vi "LSMcontroller_v63_3Dfocus.vi"() -> ()   [LabVIEW 2015] (continued)
                                n2570 = Bundle By Name(cluster=w5649, "AO"=w5648, "E_AO"=w5647) -> (w5646:T25)
                                n2571 = call "tempconfigAO.vi"("Temp Config in"=w5646, "command"="set") -> ()  [unwired: 1 out]
                                }
                                frame #1 {
                                n2572 = call "tempconfigAI.vi"("command"="get") -> ("Temp Config out"=w5661:T26)  [unwired: 1 in]
                                n2573 = Unbundle By Name(w5661) -> ("AI"=w5666:refnum<k21>, "E_AI"=w5667:errorcluster)
                                n2574 = call <vilib>:"DAQmx Start Task.vi"("task/channels in"=w5666, "error in"=w5667) -> ("task out"=w5668:refnum<k21>, "error out"=w5669:errorcluster)  [unwired: 12 in]
                                n2575 = call "tempconfigAI.vi"("command"="get") -> ("Temp Config out"=w5663:T26)  [unwired: 1 in]
                                n2576 = Bundle By Name(cluster=w5663, "AI"=w5668, "E_AI"=w5669) -> (w5665:T26)
                                n2577 = call "tempconfigAI.vi"("Temp Config in"=w5665, "command"="set") -> ()  [unwired: 1 out]
                                }
                                }
                                }
                              }
                              n2578 = case shown="True" w5645 {
                                frame False {
                                }
                                frame True {
                                n2579 = local write "set as Rp?"(FALSE ("set as Rp?")) -> ()
                                }
                              }
                            }
                          }
                        }
                        frame True {
                        }
                      }
                      n2580 = local read "sealtest"() -> (w5526:bool)
                      n2581 = Not(x=w5526) -> (.not. x?=w5525:bool)
                    }
                  }
                  frame #4 {
                    n2582 = call "tempconfigAO.vi"("command"="get") -> ("Temp Config out"=w5696:T25)  [unwired: 1 in]
                    n2583 = Unbundle By Name(w5696) -> ("AO"=w5695:refnum<k21>[], "E_AO"=w5694:errorcluster[])
                    n2584 = call "configuration.vi"("command"="get") -> ("config out"=w5677:T11)  [unwired: 2 in, 1 out]
                    n2585 = call "tempconfigAI.vi"("command"="get") -> ("Temp Config out"=w5683:T26)  [unwired: 1 in]
                    n2586 = Unbundle By Name(w5677) -> ("Device 1 sampleclock out"=w5674:tag, "Device 1 Starttrigger out"=w5673:tag)
                    n2587 = Unbundle By Name(w5683) -> ("AI"=w5684:refnum<k21>, "E_AI"=w5685:errorcluster)
                    n2588 = for {
                      tunnel: w5695 -> [w5700] mode=indexing
                      tunnel: w5694 -> [w5699] mode=indexing
                      tunnel: [w5698] -> w5690 mode=indexing
                      n2589 = call <vilib>:"DAQmx Stop Task.vi"("task/channels in"=w5700, "error in"=w5699) -> ("task out"=w5701:refnum<k21>, "error out"=w5702:errorcluster)  [unwired: 12 in]
                      n2590 = call <vilib>:"DAQmx Clear Task.vi"("task in"=w5701, "error in"=w5702) -> ("error out"=w5698:errorcluster)  [unwired: 13 in]
                    }
                    n2591 = call <vilib>:"DAQmx Stop Task.vi"("task/channels in"=w5684, "error in"=w5685) -> ("task out"=w5681:refnum<k21>, "error out"=w5680:errorcluster)  [unwired: 12 in]
                    n2592 = call <vilib>:"DAQmx Disconnect Terminals.vi"("source terminal"=tag "/Dev1/ai/SampleClock", "destination terminal"=w5674) -> ("error out"=w5671:errorcluster)  [unwired: 13 in]
                    n2593 = call <vilib>:"DAQmx Clear Task.vi"("task in"=w5681, "error in"=w5680) -> ("error out"=w5679:errorcluster)  [unwired: 13 in]
                    n2594 = call "tempconfigAO.vi"("command"="get") -> ("Temp Config out"=w5691:T25)  [unwired: 1 in]
                    n2595 = Bundle By Name(cluster=w5691, "E_AO"=w5690) -> (w5689:T25)
                    n2596 = call "tempconfigAI.vi"("command"="get") -> ("Temp Config out"=w5687:T26)  [unwired: 1 in]
                    n2597 = Bundle By Name(cluster=w5687, "E_AI"=w5679) -> (w5678:T26)
                    n2598 = call "tempconfigAO.vi"("Temp Config in"=w5689, "command"="set") -> ()  [unwired: 1 out]
                    n2599 = call <vilib>:"DAQmx Disconnect Terminals.vi"("source terminal"=tag "/Dev1/ai/StartTrigger", "destination terminal"=w5673, "error in"=w5671) -> ()  [unwired: 12 in, 1 out]
                    n2600 = call "tempconfigAI.vi"("Temp Config in"=w5678, "command"="set") -> ()  [unwired: 1 out]
                  }
                  frame #5 {
                    w5705 = T21 4 items=["no dialog", "OK message", "continue or stop message", "OK message + warnings", "continue/stop + warnings"] ("type of dialog (OK msg:1)")
                    n2601 = call "displayerrors.vi"() -> ("error IO"=w5704:errorcluster)
                    n2602 = call "zeropatch.vi"() -> ()  [unwired: 12 in]
                    n2603 = call <vilib>:"Simple Error Handler.vi"("type of dialog (OK msg:1)"=w5705, "error in (no error)"=w5704) -> ("error out"=w5703:errorcluster)  [unwired: 3 in, 4 out]
                    n2604 = call <vilib>:"Clear Errors.vi"("error in (no error)"=w5703) -> ()  [unwired: 5 in, 2 out]
                  }
                }
              }
            }
          }
          event "readpatch": Value Change {
            n2605 = event-data() -> ()  [unwired: 1 in, 6 out]
            n2606 = local read "readpatch"() -> (w5706:bool)
            n2607 = case shown="True" w5706 {
              frame False {
              }
              frame True {
                n2608 = stacked-sequence {
                  seq-local: [w5707 _ _ _ _ _] -> [_ w5740 _ w5792 _ _]
                  frame #0 {
                    n2609 = stacked-sequence {
                      tunnel: [_ w5719 _] -> w5707
                      frame #0 {
                        n2610 = call "2pparameters.vi"("command"="get") -> ("params out"=w5712:T10)  [unwired: 1 in]
                        n2611 = Unbundle By Name(w5712) -> ("autoshutter"=w5713:bool)
                        n2612 = local read "OCchecked?"() -> (w5710:bool)
                        n2613 = call "sealtestwfparams.vi"("command"="set") -> ()  [unwired: 6 in, 1 out]
                        n2614 = case shown="False" w5710 {
                          frame False {
                            n2615 = One Button Dialog(message="Is the OC gain correct?", button name ("OK")="ok") -> (true=w5714:bool)
                            n2616 = local write "OCchecked?"(w5714) -> ()
                          }
                          frame True {
                          }
                        }
                        n2617 = case shown="True" w5713 {
                          frame False {
                          }
                          frame True {
                            n2618 = call "shuttercontrol.vi"("command"="close") -> ()  [unwired: 1 in, 1 out]
                          }
                        }
                        n2619 = call "allAI-temp.vi"("command"=enum16{"get", "set", "clear", "append"}."clear") -> ()  [unwired: 3 in, 2 out]
                      }
                      frame #1 {
                        n2620 = call "sealtestwfparams.vi"("command"="get") -> ("Params out"=w5725:T22)  [unwired: 6 in]
                        n2621 = Unbundle By Name(w5725) -> ("AO parameters"=w5723:T23)
                        n2622 = Index Array(array=w5723, index=1) -> (element=w5722:T24)
                        n2623 = call "generateRampedSquareWave_fromAOparameters.vi"("AO params"=w5722) -> ("Waveform"=w5718:waveform(dbl), "wflength"=w5719:i32)
                        n2624 = Build Array(w5718) -> (w5721:waveform(dbl)[])
                        n2625 = call "waveformssealtestbuffer.vi"("AO wf in"=w5721, "command"="set") -> ()  [unwired: 1 out]
                      }
                      frame #2 {
                        n2626 = local read "Vholding (mV)"() -> (w5728:sgl)
                        n2627 = local read "Current Clamp"() -> (w5734:bool)
                        n2628 = local read "Voltage Clamp"() -> (w5733:bool)
                        n2629 = local read "OCgain"() -> (w5729:sgl)
                        n2630 = local read "CC_ICgain"() -> (w5732:dbl)
                        n2631 = local read "holdon"() -> (w5727:bool)
                        n2632 = call "patchparameters.vi"("command"="get") -> ("Params out"=w5736:T13)  [unwired: 1 in]
                        n2633 = Bundle By Name(cluster=w5736, "VC"=w5733, "CC"=w5734, "CC_icg (pA/mv)"=w5732, "VC_icg (mV/mV)"=10.0, "OCG (mV/pA)"=w5729, "OVG (mV/mV)"=0.1, "Vhold (mV)"=w5728, "holdon"=w5727) -> (w5735:T13)
                        n2634 = call "patchparameters.vi"("Params in"=w5735, "command"="set") -> ()  [unwired: 1 out]
                      }
                    }
                  }
                  frame #1 {
                    w5739 = 2
                    n2635 = call "patchparameters.vi"("command"="get") -> ("Params out"=w5747:T13)  [unwired: 1 in]
                    n2636 = Unbundle By Name(w5747) -> ("holdon"=w5746:bool, "Vhold (mV)"=w5745:sgl, "CC_icg (pA/mv)"=w5753:sgl, "CC"=w5751:bool, "VC_icg (mV/mV)"=w5752:sgl)
                    n2637 = Select(t=w5753, s=w5751, f=w5752) -> (s? t:f=w5754:sgl)
                    n2638 = To Single Precision Float(number=0.001 ("y")) -> (single precision float=w5755:sgl)
                    n2639 = Compound Arithmetic op=MULTIPLY(w5745, w5754, w5755) -> (w5749:sgl)
                    n2640 = case shown="False" w5746 {
                      tunnel: w5749 -> [_ w5767]
                      tunnel: [0.0 w5767] -> w5742
                      frame False {
                      }
                      frame True {
                      }
                    }
                    n2641 = Greater Than 0?(x=w5739) -> (x > 0?=w5741:bool)
                    n2642 = case shown="True" w5741 {
                      tunnel: w5740 -> [_ w5756]
                      tunnel: w5739 -> [_ w5759]
                      frame False {
                      }
                      frame True {
                        n2643 = Initialize Array(sgl 0.0 ("element"), w5759, w5756) -> (w5757:sgl[][])
                        n2644 = call "allAI-temp.vi"("array in"=w5757, "command"=enum16{"get", "set", "clear", "append"}."set") -> ()  [unwired: 2 in, 2 out]
                      }
                    }
                    n2645 = flat-sequence {
                      tunnel: w5740 -> [w5763]
                      tunnel: w5740 -> [w5762]
                      tunnel: [w5762] -> w5744
                      tunnel: [w5761] -> w5743
                      tunnel: w5742 -> [w5761]
                      tunnel: w5744 -> [w5765]
                      tunnel: w5743 -> [w5764]
                      frame #0 {
                        n2646 = call "prepAI_sealtest.vi"("samples per channel"=w5763) -> ()  [unwired: 2 in]
                      }
                      frame #1 {
                        n2647 = call "prepAO_sealtest.vi"("Vhold"=w5764, "samples per channel"=w5765) -> ()  [unwired: 1 in]
                      }
                    }
                  }
                  frame #2 {
                    n2648 = stacked-sequence {
                      frame #0 {
                        n2649 = call "tempconfigAO.vi"("command"="get") -> ("Temp Config out"=w5771:T25)  [unwired: 1 in]
                        n2650 = Unbundle By Name(w5771) -> ("AO"=w5772:refnum<k21>[], "E_AO"=w5773:errorcluster[])
                        n2651 = for {
                          tunnel: w5772 -> [w5781] mode=indexing
                          tunnel: w5773 -> [w5780] mode=indexing
                          tunnel: [w5779] -> w5775 mode=indexing
                          tunnel: [w5778] -> w5776 mode=indexing
                          n2652 = call <vilib>:"DAQmx Start Task.vi"("task/channels in"=w5781, "error in"=w5780) -> ("task out"=w5779:refnum<k21>, "error out"=w5778:errorcluster)  [unwired: 12 in]
                        }
                        n2653 = call "tempconfigAO.vi"("command"="get") -> ("Temp Config out"=w5774:T25)  [unwired: 1 in]
                        n2654 = Bundle By Name(cluster=w5774, "AO"=w5775, "E_AO"=w5776) -> (w5777:T25)
                        n2655 = call "tempconfigAO.vi"("Temp Config in"=w5777, "command"="set") -> ()  [unwired: 1 out]
                      }
                      frame #1 {
                        n2656 = call "tempconfigAI.vi"("command"="get") -> ("Temp Config out"=w5783:T26)  [unwired: 1 in]
                        n2657 = Unbundle By Name(w5783) -> ("AI"=w5788:refnum<k21>, "E_AI"=w5789:errorcluster)
                        n2658 = call <vilib>:"DAQmx Start Task.vi"("task/channels in"=w5788, "error in"=w5789) -> ("task out"=w5790:refnum<k21>, "error out"=w5791:errorcluster)  [unwired: 12 in]
                        n2659 = call "tempconfigAI.vi"("command"="get") -> ("Temp Config out"=w5785:T26)  [unwired: 1 in]
                        n2660 = Bundle By Name(cluster=w5785, "AI"=w5790, "E_AI"=w5791) -> (w5787:T26)
                        n2661 = call "tempconfigAI.vi"("Temp Config in"=w5787, "command"="set") -> ()  [unwired: 1 out]
                      }
                    }
                  }
                  frame #3 {
                    n2662 = while {
                      tunnel: w5792 -> [w5793]
                      stop <- w5794 stop-if-true
                      n2663 = local read "readpatch"() -> (w5797:bool)
                      n2664 = Not(x=w5797) -> (.not. x?=w5796:bool)
                      n2665 = case shown="True" w5796 {
                        tunnel: w5793 -> [w5798 _]
                        frame False {
                          n2666 = stacked-sequence {
                            seq-local: [w5799 _ _ _ _ _] -> [_ w5808 _ w5831 w5878 w5897]
                            tunnel: w5798 -> [_ _ w5816 _ w5877 _]
                            frame #0 {
                              n2667 = call "patchparameters.vi"("command"="get") -> ("Params out"=w5806:T13)  [unwired: 1 in]
                              n2668 = local read "Vholding (mV)"() -> (w5803:sgl)
                              n2669 = Unbundle By Name(w5806) -> ("Vhold (mV)"=w5802:sgl, "holdon"=w5805:bool)
                              n2670 = local read "holdon"() -> (w5804:bool)
                              n2671 = Not Equal?(x=w5803, y=w5802) -> (x != y?=w5801:bool)
                              n2672 = Not Equal?(x=w5805, y=w5804) -> (x != y?=w5800:bool)
                              n2673 = Or(x=w5801, y=w5800) -> (x .or. y?=w5799:bool)
                            }
                            frame #1 {
                              n2674 = case shown="False" w5808 {
                                frame False {
                                }
                                frame True {
                                n2675 = local read "Vholding (mV)"() -> (w5811:sgl)
                                n2676 = local read "holdon"() -> (w5809:bool)
                                n2677 = call "patchparameters.vi"("command"="get") -> ("Params out"=w5812:T13)  [unwired: 1 in]
                                n2678 = Bundle By Name(cluster=w5812, "Vhold (mV)"=w5811, "holdon"=w5809) -> (w5810:T13)
                                n2679 = call "patchparameters.vi"("Params in"=w5810, "command"="set") -> ()  [unwired: 1 out]
                                }
                              }
                            }
                            frame #2 {
                              n2680 = call "tempconfigAI.vi"("command"="get") -> ("Temp Config out"=w5826:T26)  [unwired: 1 in]
                              n2681 = Unbundle By Name(w5826) -> ("AI"=w5825:refnum<k21>, "E_AI"=w5824:errorcluster)
                              n2682 = call-poly <vilib>:"DAQmx Read.vi"("task/channels in"=w5825, "number of samples per channel"=w5816, "timeout"=10.0, "error in"=w5824) -> ("task out"=w5820:refnum<k21>, "data"=w5817:i16[][], "error out"=w5829:errorcluster)  [unwired: 9 in]
                              n2683 = call "tempconfigAI.vi"("command"="get") -> ("Temp Config out"=w5821:T26)  [unwired: 1 in]
                              n2684 = Bundle By Name(cluster=w5821, "AI"=w5820, "E_AI"=w5829) -> (w5828:T26)
                              n2685 = To Single Precision Float(number=w5817) -> (single precision float=w5819:sgl[][])
                              n2686 = call "tempconfigAI.vi"("Temp Config in"=w5828, "command"="set") -> ()  [unwired: 1 out]
                              n2687 = call "allAI-temp.vi"("array in"=w5819, "command"=enum16{"get", "set", "clear", "append"}."set") -> ()  [unwired: 2 in, 2 out]
                            }
                            frame #3 {
                              n2688 = case shown="True" w5831 {
                                frame False {
                                }
                                frame True {
                                n2689 = call "tempconfigAO.vi"("command"="get") -> ("Temp Config out"=w5870:T25)  [unwired: 1 in]
                                n2690 = Unbundle By Name(w5870) -> ("AO"=w5869:refnum<k21>[], "E_AO"=w5868:errorcluster[])
                                n2691 = call "tempconfigAI.vi"("command"="get") -> ("Temp Config out"=w5857:T26)  [unwired: 1 in]
                                n2692 = Unbundle By Name(w5857) -> ("AI"=w5858:refnum<k21>, "E_AI"=w5859:errorcluster)
                                n2693 = for {
                                tunnel: w5869 -> [w5874] mode=indexing
                                tunnel: w5868 -> [w5873] mode=indexing
                                tunnel: [w5872] -> w5864 mode=indexing
                                n2694 = call <vilib>:"DAQmx Stop Task.vi"("task/channels in"=w5874, "error in"=w5873) -> ("task out"=w5875:refnum<k21>, "error out"=w5876:errorcluster)  [unwired: 12 in]
                                n2695 = call <vilib>:"DAQmx Clear Task.vi"("task in"=w5875, "error in"=w5876) -> ("error out"=w5872:errorcluster)  [unwired: 13 in]
                                }
                                n2696 = call <vilib>:"DAQmx Stop Task.vi"("task/channels in"=w5858, "error in"=w5859) -> ("task out"=w5855:refnum<k21>, "error out"=w5854:errorcluster)  [unwired: 12 in]
                                n2697 = call <vilib>:"DAQmx Clear Task.vi"("task in"=w5855, "error in"=w5854) -> ("error out"=w5853:errorcluster)  [unwired: 13 in]
                                n2698 = call "tempconfigAO.vi"("command"="get") -> ("Temp Config out"=w5865:T25)  [unwired: 1 in]
                                n2699 = Bundle By Name(cluster=w5865, "E_AO"=w5864) -> (w5863:T25)
                                n2700 = call "tempconfigAI.vi"("command"="get") -> ("Temp Config out"=w5861:T26)  [unwired: 1 in]
                                n2701 = Bundle By Name(cluster=w5861, "E_AI"=w5853) -> (w5852:T26)
                                n2702 = call "tempconfigAO.vi"("Temp Config in"=w5863, "command"="set") -> ()  [unwired: 1 out]
                                n2703 = call "tempconfigAI.vi"("Temp Config in"=w5852, "command"="set") -> ()  [unwired: 1 out]
                                }
                              }
                              n2704 = call "allAI-temp.vi"("command"=enum16{"get", "set", "clear", "append"}."get") -> ("array out"=w5835:sgl[][])  [unwired: 3 in, 1 out]
                              n2705 = call "tempconfigAI.vi"("command"="get") -> ("Temp Config out"=w5847:T26)  [unwired: 1 in]
                              n2706 = call "tempconfigAI.vi"("command"="get") -> ("Temp Config out"=w5849:T26)  [unwired: 1 in]
                              n2707 = Unbundle By Name(w5847) -> ("header"=w5845:dbl[])
                              n2708 = Unbundle By Name(w5849) -> ("header"=w5851:dbl[])
                              n2709 = Index Array(array=w5835, index (row) #1=1 ("index (row)"), index (row) #2=0 ("index (row)")) -> (element #1=w5833:sgl[], element #2=w5832:sgl[])  [unwired: 2 in]
                              n2710 = local read "OCgain"() -> (w5839:sgl)
                              n2711 = call "Unscaledtoscaled.vi"("Unscaled Data"=w5833, "Header Information"=w5845) -> ("Array"=w5844:sgl[])  [unwired: 1 in]
                              n2712 = call "Unscaledtoscaled.vi"("Unscaled Data"=w5832, "Header Information"=w5851) -> ("Array"=w5848:sgl[])  [unwired: 1 in]
                              n2713 = Multiply(x=w5844, y=0.1) -> (x*y=w5841:dbl[])
                              n2714 = Divide(x=w5848, y=w5839) -> (x/y=w5840:sgl[])
                              n2715 = Build Array(w5841, w5840) -> (w5843:dbl[][])
                              n2716 = Multiply(x=w5843, y=1000.0) -> (x*y=w5830:dbl[][])
                              n2717 = local write "Patch readout"(w5830) -> ()
                            }
                            frame #4 {
                              n2718 = case shown="True" w5878 {
                                tunnel: w5877 -> [_ w5879]
                                frame False {
                                }
                                frame True {
                                n2719 = call "patchparameters.vi"("command"="get") -> ("Params out"=w5883:T13)  [unwired: 1 in]
                                n2720 = Unbundle By Name(w5883) -> ("holdon"=w5882:bool, "Vhold (mV)"=w5881:sgl, "CC_icg (pA/mv)"=w5889:sgl, "CC"=w5887:bool, "VC_icg (mV/mV)"=w5888:sgl)
                                n2721 = Select(t=w5889, s=w5887, f=w5888) -> (s? t:f=w5890:sgl)
                                n2722 = To Single Precision Float(number=0.001 ("y")) -> (single precision float=w5891:sgl)
                                n2723 = Compound Arithmetic op=MULTIPLY(w5881, w5890, w5891) -> (w5885:sgl)
                                n2724 = case shown="True" w5882 {
                                tunnel: w5885 -> [_ w5896]
                                tunnel: [0.0 w5896] -> w5880
                                frame False {
                                }
                                frame True {
                                }
                                }
                                n2725 = flat-sequence {
                                tunnel: w5879 -> [w5892]
                                tunnel: w5880 -> [w5894]
                                tunnel: w5879 -> [w5893]
                                frame #0 {
                                n2726 = call "prepAI_sealtest.vi"("samples per channel"=w5892) -> ()  [unwired: 2 in]
                                }
                                frame #1 {
                                n2727 = call "prepAO_sealtest.vi"("Vhold"=w5894, "samples per channel"=w5893) -> ()  [unwired: 1 in]
                                }
                                }
                                }
                              }
                            }
                            frame #5 {
                              n2728 = case shown="True" w5897 {
                                frame False {
                                }
                                frame True {
                                n2729 = stacked-sequence {
                                frame #0 {
                                n2730 = call "tempconfigAO.vi"("command"="get") -> ("Temp Config out"=w5904:T25)  [unwired: 1 in]
                                n2731 = Unbundle By Name(w5904) -> ("AO"=w5903:refnum<k21>[], "E_AO"=w5902:errorcluster[])
                                n2732 = for {
                                tunnel: w5903 -> [w5911] mode=indexing
                                tunnel: w5902 -> [w5910] mode=indexing
                                tunnel: [w5909] -> w5900 mode=indexing
                                tunnel: [w5908] -> w5899 mode=indexing
                                n2733 = call <vilib>:"DAQmx Start Task.vi"("task/channels in"=w5911, "error in"=w5910) -> ("task out"=w5909:refnum<k21>, "error out"=w5908:errorcluster)  [unwired: 12 in]
                                }
                                n2734 = call "tempconfigAO.vi"("command"="get") -> ("Temp Config out"=w5901:T25)  [unwired: 1 in]
                                n2735 = Bundle By Name(cluster=w5901, "AO"=w5900, "E_AO"=w5899) -> (w5898:T25)
                                n2736 = call "tempconfigAO.vi"("Temp Config in"=w5898, "command"="set") -> ()  [unwired: 1 out]
                                }
                                frame #1 {
                                n2737 = call "tempconfigAI.vi"("command"="get") -> ("Temp Config out"=w5913:T26)  [unwired: 1 in]
                                n2738 = Unbundle By Name(w5913) -> ("AI"=w5918:refnum<k21>, "E_AI"=w5919:errorcluster)
                                n2739 = call <vilib>:"DAQmx Start Task.vi"("task/channels in"=w5918, "error in"=w5919) -> ("task out"=w5920:refnum<k21>, "error out"=w5921:errorcluster)  [unwired: 12 in]
                                n2740 = call "tempconfigAI.vi"("command"="get") -> ("Temp Config out"=w5915:T26)  [unwired: 1 in]
                                n2741 = Bundle By Name(cluster=w5915, "AI"=w5920, "E_AI"=w5921) -> (w5917:T26)
                                n2742 = call "tempconfigAI.vi"("Temp Config in"=w5917, "command"="set") -> ()  [unwired: 1 out]
                                }
                                }
                                }
                              }
                            }
                          }
                        }
                        frame True {
                        }
                      }
                      n2743 = local read "readpatch"() -> (w5795:bool)
                      n2744 = Not(x=w5795) -> (.not. x?=w5794:bool)
                    }
                  }
                  frame #4 {
                    n2745 = call "tempconfigAO.vi"("command"="get") -> ("Temp Config out"=w5947:T25)  [unwired: 1 in]
                    n2746 = Unbundle By Name(w5947) -> ("AO"=w5946:refnum<k21>[], "E_AO"=w5945:errorcluster[])
                    n2747 = call "configuration.vi"("command"="get") -> ("config out"=w5928:T11)  [unwired: 2 in, 1 out]
                    n2748 = call "tempconfigAI.vi"("command"="get") -> ("Temp Config out"=w5934:T26)  [unwired: 1 in]
                    n2749 = Unbundle By Name(w5928) -> ("Device 1 sampleclock out"=w5925:tag, "Device 1 Starttrigger out"=w5924:tag)
                    n2750 = Unbundle By Name(w5934) -> ("AI"=w5935:refnum<k21>, "E_AI"=w5936:errorcluster)
                    n2751 = for {
                      tunnel: w5946 -> [w5951] mode=indexing
                      tunnel: w5945 -> [w5950] mode=indexing
                      tunnel: [w5949] -> w5941 mode=indexing
                      n2752 = call <vilib>:"DAQmx Stop Task.vi"("task/channels in"=w5951, "error in"=w5950) -> ("task out"=w5952:refnum<k21>, "error out"=w5953:errorcluster)  [unwired: 12 in]
                      n2753 = call <vilib>:"DAQmx Clear Task.vi"("task in"=w5952, "error in"=w5953) -> ("error out"=w5949:errorcluster)  [unwired: 13 in]
                    }
                    n2754 = call <vilib>:"DAQmx Stop Task.vi"("task/channels in"=w5935, "error in"=w5936) -> ("task out"=w5932:refnum<k21>, "error out"=w5931:errorcluster)  [unwired: 12 in]
                    n2755 = call <vilib>:"DAQmx Disconnect Terminals.vi"("source terminal"=tag "/Dev1/ai/SampleClock", "destination terminal"=w5925) -> ("error out"=w5922:errorcluster)  [unwired: 13 in]
                    n2756 = call <vilib>:"DAQmx Clear Task.vi"("task in"=w5932, "error in"=w5931) -> ("error out"=w5930:errorcluster)  [unwired: 13 in]
                    n2757 = call "tempconfigAO.vi"("command"="get") -> ("Temp Config out"=w5942:T25)  [unwired: 1 in]
                    n2758 = Bundle By Name(cluster=w5942, "E_AO"=w5941) -> (w5940:T25)
                    n2759 = call "tempconfigAI.vi"("command"="get") -> ("Temp Config out"=w5938:T26)  [unwired: 1 in]
                    n2760 = Bundle By Name(cluster=w5938, "E_AI"=w5930) -> (w5929:T26)
                    n2761 = call "tempconfigAO.vi"("Temp Config in"=w5940, "command"="set") -> ()  [unwired: 1 out]
                    n2762 = call <vilib>:"DAQmx Disconnect Terminals.vi"("source terminal"=tag "/Dev1/ai/StartTrigger", "destination terminal"=w5924, "error in"=w5922) -> ()  [unwired: 12 in, 1 out]
                    n2763 = call "tempconfigAI.vi"("Temp Config in"=w5929, "command"="set") -> ()  [unwired: 1 out]
                  }
                  frame #5 {
                    w5956 = T21 4 items=["no dialog", "OK message", "continue or stop message", "OK message + warnings", "continue/stop + warnings"] ("type of dialog (OK msg:1)")
                    n2764 = call "displayerrors.vi"() -> ("error IO"=w5955:errorcluster)
                    n2765 = call "zeropatch.vi"() -> ()  [unwired: 12 in]
                    n2766 = call <vilib>:"Simple Error Handler.vi"("type of dialog (OK msg:1)"=w5956, "error in (no error)"=w5955) -> ("error out"=w5954:errorcluster)  [unwired: 3 in, 4 out]
                    n2767 = call <vilib>:"Clear Errors.vi"("error in (no error)"=w5954) -> ()  [unwired: 5 in, 2 out]
                  }
                }
              }
            }
          }
          event "Current Clamp": Value Change {
            n2768 = event-data() -> ()  [unwired: 1 in, 6 out]
            n2769 = local read "Current Clamp"() -> (w5961:bool)
            n2770 = property on="Vholding (mV)" class="DigNum (strict)"("Caption.Text"="Ihold (pA)") -> ()  [unwired: 2 in, 2 out]
            n2771 = Not(x=w5961) -> (.not. x?=w5960:bool)
            n2772 = property on="Voltage Clamp" class="Bool (strict)"("Value"=w5960) -> ()  [unwired: 2 in, 2 out]
            n2773 = One Button Dialog(message="Have you switched the HEKA to CC and changed the external input cable?", button name ("OK")="Ok") -> ()  [unwired: 1 out]
          }
          event "Voltage Clamp": Value Change {
            n2774 = event-data() -> ()  [unwired: 1 in, 6 out]
            n2775 = local read "Voltage Clamp"() -> (w5966:bool)
            n2776 = Not(x=w5966) -> (.not. x?=w5965:bool)
            n2777 = property on="Current Clamp" class="Bool (strict)"("Value"=w5965) -> ()  [unwired: 2 in, 2 out]
            n2778 = One Button Dialog(message="Have you switched the HEKA to VC and changed the external input cable?", button name ("OK")="Ok") -> ()  [unwired: 1 out]
            n2779 = property on="Vholding (mV)" class="DigNum (strict)"("Caption.Text"="Vhold (mV)") -> ()  [unwired: 2 in, 2 out]
          }
          event "OCgain": Value Change {
            n2780 = event-data() -> ()  [unwired: 1 in, 6 out]
            n2781 = local read "OCgain"() -> (w5969:sgl)
            n2782 = Less?(x=w5969, y=0.3) -> (x < y?=w5967:bool)
            n2783 = case shown="True" w5967 {
              frame False {
                w5970 = 10.0 items=["0.1"=10.0, "10"=0.1] ("CC_ICgain")
                n2784 = local write "CC_ICgain"(w5970) -> ()
              }
              frame True {
                w5971 = 0.1 items=["0.1"=10.0, "10"=0.1] ("CC_ICgain")
                n2785 = local write "CC_ICgain"(w5971) -> ()
              }
            }
          }
          event "holdon": Value Change {
            n2786 = event-data() -> ()  [unwired: 1 in, 6 out]
            n2787 = stacked-sequence {
              frame #0 {
                n2788 = local read "Vholding (mV)"() -> (w5975:sgl)
                n2789 = local read "holdon"() -> (w5972:bool)
                n2790 = call "patchparameters.vi"("command"="get") -> ("Params out"=w5976:T13)  [unwired: 1 in]
                n2791 = Bundle By Name(cluster=w5976, "Vhold (mV)"=w5975, "holdon"=w5972) -> (w5973:T13)
                n2792 = call "patchparameters.vi"("Params in"=w5973, "command"="set") -> ()  [unwired: 1 out]
              }
              frame #1 {
                n2793 = call "zeropatch.vi"() -> ()  [unwired: 12 in]
              }
            }
          }
          event "Vholding (mV)": Value Change {
            n2794 = event-data() -> ()  [unwired: 1 in, 6 out]
            n2795 = local read "holdon"() -> (w5978:bool)
            n2796 = case shown="True" w5978 {
              frame False {
              }
              frame True {
                n2797 = stacked-sequence {
                  frame #0 {
                    n2798 = local read "Vholding (mV)"() -> (w5981:sgl)
                    n2799 = local read "holdon"() -> (w5982:bool)
                    n2800 = call "patchparameters.vi"("command"="get") -> ("Params out"=w5983:T13)  [unwired: 1 in]
                    n2801 = Bundle By Name(cluster=w5983, "Vhold (mV)"=w5981, "holdon"=w5982) -> (w5979:T13)
                    n2802 = call "patchparameters.vi"("Params in"=w5979, "command"="set") -> ()  [unwired: 1 out]
                  }
                  frame #1 {
                    n2803 = call "zeropatch.vi"() -> ()  [unwired: 12 in]
                  }
                }
              }
            }
          }
          event "AI channels": Value Change {
            n2804 = event-data() -> ()  [unwired: 1 in, 6 out]
            n2805 = local read "CI channels"() -> (w5992:i32[])
            n2806 = local read "AI channels"() -> (w5993:i32[])
            n2807 = call "configuration.vi"("command"="get") -> ("config out"=w5986:T11)  [unwired: 2 in, 1 out]
            n2808 = Unbundle By Name(w5986) -> ("CI names"=w5987:string[], "AI names"=w5988:string[])
            n2809 = for {
              tunnel: w5992 -> [w5998] mode=indexing
              tunnel: w5987 -> [w5999]
              tunnel: [w5997] -> w5989 mode=indexing
              n2810 = Index Array(array=w5999, index=w5998) -> (element=w5997:string)
            }
            n2811 = for {
              tunnel: w5993 -> [w5995] mode=indexing
              tunnel: w5988 -> [w5996]
              tunnel: [w5994] -> w5990 mode=indexing
              n2812 = Index Array(array=w5996, index=w5995) -> (element=w5994:string)
            }
            n2813 = Build Array (concatenate)(w5989, w5990) -> (w5991:string[])
            n2814 = property on="image1list" class="Ring (strict)"("Strings []"=w5991) -> ()  [unwired: 2 in, 2 out]
            n2815 = property on="image2list" class="Ring (strict)"("Strings []"=w5991) -> ()  [unwired: 2 in, 2 out]
          }
          event "CI channels": Value Change {
            n2816 = event-data() -> ()  [unwired: 1 in, 6 out]
            n2817 = local read "CI channels"() -> (w6007:i32[])
            n2818 = local read "AI channels"() -> (w6008:i32[])
            n2819 = call "configuration.vi"("command"="get") -> ("config out"=w6001:T11)  [unwired: 2 in, 1 out]
            n2820 = Unbundle By Name(w6001) -> ("CI names"=w6002:string[], "AI names"=w6003:string[])
            n2821 = for {
              tunnel: w6007 -> [w6013] mode=indexing
              tunnel: w6002 -> [w6014]
              tunnel: [w6012] -> w6004 mode=indexing
              n2822 = Index Array(array=w6014, index=w6013) -> (element=w6012:string)
            }
            n2823 = for {
              tunnel: w6008 -> [w6010] mode=indexing
              tunnel: w6003 -> [w6011]
              tunnel: [w6009] -> w6005 mode=indexing
              n2824 = Index Array(array=w6011, index=w6010) -> (element=w6009:string)
            }
            n2825 = Build Array (concatenate)(w6004, w6005) -> (w6006:string[])
            n2826 = property on="image1list" class="Ring (strict)"("Strings []"=w6006) -> ()  [unwired: 2 in, 2 out]
            n2827 = property on="image2list" class="Ring (strict)"("Strings []"=w6006) -> ()  [unwired: 2 in, 2 out]
          }
          event "setdatdir": Value Change {
            n2828 = event-data() -> ()  [unwired: 1 in, 5 out]
            n2829 = case shown="True" "setdatdir" {
              frame False {
              }
              frame True {
                n2830 = stacked-sequence {
                  frame #0 {
                    n2831 = local read "data dir"() -> (w6016:path)
                    n2832 = call "File Dialog"("start path"=w6016, "prompt"="Please select data directory...") -> ("selected path"=w6018:path, "cancelled"=w6017:bool, "error out"=w6019:errorcluster)  [unwired: 10 in, 1 out]
                    n2833 = case shown="False" w6017 {
                      tunnel: w6018 -> [w6027 _]
                      tunnel: w6019 -> [w6024 w6030]
                      tunnel: [w6022 w6030] -> w6021
                      frame False {
                        n2834 = local write "data dir"(w6027) -> ()
                        n2835 = call "configuration.vi"("error in"=w6024, "command"="get") -> ("Error out"=w6023:errorcluster, "config out"=w6029:T11)  [unwired: 1 in]
                        n2836 = Bundle By Name(cluster=w6029, "master data dir"=w6027) -> (w6028:T11)
                        n2837 = call "configuration.vi"("error in"=w6023, "config in"=w6028, "command"="set") -> ("Error out"=w6022:errorcluster)  [unwired: 1 out]
                      }
                      frame True {
                      }
                    }
                    n2838 = local write "status"(w6021) -> ()
                  }
                  frame #1 {
                    n2839 = property on="setdatdir" class="Bool (strict)"("Value"=FALSE ("setdatdir")) -> ()  [unwired: 2 in, 2 out]
                  }
                }
              }
            }
          }
          event "Shutter": Value Change {
            n2840 = event-data() -> ()  [unwired: 1 in, 5 out]
            n2841 = case shown="False" "Shutter" {
              frame False {
                n2842 = call "shuttercontrol.vi"("command"="close") -> ()  [unwired: 1 in, 1 out]
              }
              frame True {
                n2843 = call "shuttercontrol.vi"("command"="open") -> ()  [unwired: 1 in, 1 out]
              }
            }
          }
          event "ROI": Value Change {
            n2844 = event-data() -> ()  [unwired: 1 in, 5 out]
            n2845 = local read "ROI"() -> (w6035:bool)
            n2846 = case shown="True" w6035 {
              frame False {
              }
              frame True {
                n2847 = stacked-sequence {
                  frame #0 {
                    n2848 = local read "Square pixels"() -> (w6052:bool)
                    n2849 = local read "square matrix"() -> (w6051:bool)
                    n2850 = local read "Vx-max ref"() -> (w6057:dbl)
                    n2851 = local read "Vx-min ref"() -> (w6056:dbl)
                    n2852 = local read "Vy-min ref"() -> (w6053:dbl)
                    n2853 = local read "ypixels ref"() -> (w6055:i32)
                    n2854 = local read "Vy-max ref"() -> (w6054:dbl)
                    n2855 = local read "xpixels ref"() -> (w6058:i32)
                    n2856 = local read "Angle ref"() -> (w6050:dbl)
                    n2857 = local read "Colormap"() -> (w6059:i32)
                    n2858 = call "2pparameters.vi"("command"="get") -> ("params out"=w6062:T10)  [unwired: 1 in]
                    n2859 = Bundle By Name(cluster=w6062, "Xpixels Img"=w6058, "Vx-min Img"=w6056, "VX-max Img"=w6057, "Ypixels Img"=w6055, "Vy-min Img"=w6053, "Vy-max Img"=w6054, "Colormap"=w6059, "square pixels"=w6052, "square matrix"=w6051, "Angle Img"=w6050) -> (w6061:T10)
                    n2860 = call "2pparameters.vi"("Params in"=w6061, "command"="set") -> ()  [unwired: 1 out]
                    n2861 = local read "Vx-max draw"() -> (w6042:dbl)
                    n2862 = local read "Angle drawing"() -> (w6049:dbl)
                    n2863 = local read "Vx-min draw"() -> (w6043:dbl)
                    n2864 = local read "Vy-min draw"() -> (w6046:dbl)
                    n2865 = local read "ypixels draw"() -> (w6044:dbl)
                    n2866 = local read "Vy-max draw"() -> (w6045:dbl)
                    n2867 = local read "Square pixels"() -> (w6047:bool)
                    n2868 = local read "square matrix"() -> (w6048:bool)
                    n2869 = local read "xpixels draw"() -> (w6041:dbl)
                    n2870 = local read "Colormap"() -> (w6040:i32)
                    n2871 = call "2pparameters.vi"("command"="get") -> ("params out"=w6037:T10)  [unwired: 1 in]
                    n2872 = Bundle By Name(cluster=w6037, "Xpixels"=w6041, "Vxminref"=w6043, "Vxmaxref"=w6042, "Ypixels"=w6044, "Vyminref"=w6046, "Vymaxref"=w6045, "Colormap"=w6040, "square pixels"=w6047, "square matrix"=w6048, "Angle draw"=w6049) -> (w6038:T10)
                    n2873 = call "2pparameters.vi"("Params in"=w6038, "command"="set") -> ()  [unwired: 1 out]
                  }
                  frame #1 {
                    n2874 = Current VI's Path() -> (path=w6073:path)
                    n2875 = Strip Path(path=w6073) -> (stripped path=w6074:path)  [unwired: 1 out]
                    n2876 = Build Path(base path=w6074, name or relative path="subVIs\\Image\\SetROI_v4.vi") -> (appended path=w6072:path)
                    n2877 = call <vilib>:"Set Busy.vi"() -> ("error out"=w6070:errorcluster)  [unwired: 10 in, 1 out]
                    n2878 = Open VI Reference(type specifier VI Refnum (for type only)=refnum<vi> refnum, vi path=w6072, error in (no error)=w6070) -> (vi reference=w6068:refnum<vi>, error out=w6066:errorcluster)  [unwired: 3 in]
                    n2879 = call-by-ref "?"(reference=w6068, error in=w6066) -> (reference out=w6067:refnum<vi>, error out=w6065:errorcluster)  [unwired: 1 in]
                    n2880 = Close Reference(reference=w6067, error in (no error)=w6065) -> (error out=w6069:errorcluster)
                    n2881 = call <vilib>:"Unset Busy.vi"("error in (no error)"=w6069) -> ()  [unwired: 10 in, 1 out]
                    n2882 = local write "status"(w6069) -> ()
                  }
                  frame #2 {
                    n2883 = call "2pparameters.vi"("command"="get") -> ("params out"=w6099:T10)  [unwired: 1 in]
                    n2884 = Unbundle By Name(w6099) -> ("Xpixels Img"=w6098:i32, "Vx-min Img"=w6097:dbl, "VX-max Img"=w6096:dbl, "Ypixels Img"=w6095:i32, "Vy-min Img"=w6094:dbl, "Vy-max Img"=w6093:dbl, "Colormap"=w6092:u16, "square pixels"=w6091:bool, "square matrix"=w6090:bool, "Angle Img"=w6089:dbl, "Drawing Mode"=w6088:u16)
                    n2885 = local write "xpixels ref"(w6098) -> ()
                    n2886 = local write "Vx-min ref"(w6097) -> ()
                    n2887 = local write "Vx-max ref"(w6096) -> ()
                    n2888 = local write "ypixels ref"(w6095) -> ()
                    n2889 = local write "Vy-min ref"(w6094) -> ()
                    n2890 = local write "Vy-max ref"(w6093) -> ()
                    n2891 = local write "Colormap"(w6092) -> ()
                    n2892 = local write "Square pixels"(w6091) -> ()
                    n2893 = local write "square matrix"(w6090) -> ()
                    n2894 = local write "Angle ref"(w6089) -> ()
                    n2895 = local write "ROI Type"(w6088) -> ()
                    n2896 = call "2pparameters.vi"("command"="get") -> ("params out"=w6082:T10)  [unwired: 1 in]
                    n2897 = Unbundle By Name(w6082) -> ("Xpixels"=w6076:i32, "Vxminref"=w6080:dbl, "Vxmaxref"=w6079:dbl, "Ypixels"=w6075:i32, "Vyminref"=w6078:dbl, "Vymaxref"=w6077:dbl, "Colormap"=w6083:u16, "square pixels"=w6084:bool, "square matrix"=w6085:bool, "Angle draw"=w6086:dbl, "Drawing Mode"=w6087:u16)
                    n2898 = local write "Vy-max draw"(w6077) -> ()
                    n2899 = local write "Angle drawing"(w6086) -> ()
                    n2900 = local write "Colormap"(w6083) -> ()
                    n2901 = local write "Square pixels"(w6084) -> ()
                    n2902 = local write "square matrix"(w6085) -> ()
                    n2903 = local write "ROI Type"(w6087) -> ()
                    n2904 = local write "xpixels draw"(w6076) -> ()
                    n2905 = local write "ypixels draw"(w6075) -> ()
                    n2906 = local write "Vx-min draw"(w6080) -> ()
                    n2907 = local write "Vx-max draw"(w6079) -> ()
                    n2908 = local write "Vy-min draw"(w6078) -> ()
                  }
                  frame #3 {
                    n2909 = property on="ROI" class="Bool (strict)"("Val(Sgnl)"=FALSE ("x/y scan")) -> ()  [unwired: 2 in, 2 out]
                  }
                }
              }
            }
          }
          event "Xdattype": Value Change {
            n2910 = event-data() -> ()  [unwired: 1 in, 1 out]
            n2911 = case shown="True" "Xdattype" {
              frame False {
              }
              frame True {
                n2912 = stacked-sequence {
                  frame #0 {
                    n2913 = Current VI's Path() -> (path=w6112:path)
                    n2914 = Strip Path(path=w6112) -> (stripped path=w6113:path)  [unwired: 1 out]
                    n2915 = Build Path(base path=w6113, name or relative path="subVIs\\Misc\\Changedataconfig.vi") -> (appended path=w6111:path)
                    n2916 = call <vilib>:"Set Busy.vi"() -> ("error out"=w6109:errorcluster)  [unwired: 10 in, 1 out]
                    n2917 = Open VI Reference(type specifier VI Refnum (for type only)=refnum<vi> refnum, vi path=w6111, error in (no error)=w6109) -> (vi reference=w6104:refnum<vi>, error out=w6106:errorcluster)  [unwired: 3 in]
                    n2918 = call-by-ref "?"(reference=w6104, error in=w6106) -> (reference out=w6108:refnum<vi>, error out=w6107:errorcluster)  [unwired: 12 in]
                    n2919 = Close Reference(reference=w6108, error in (no error)=w6107) -> (error out=w6103:errorcluster)
                    "status" <- w6103
                    n2920 = call <vilib>:"Unset Busy.vi"("error in (no error)"=w6103) -> ()  [unwired: 10 in, 1 out]
                  }
                  frame #1 {
                    n2921 = property on="Xdattype" class="Bool (strict)"("Val(Sgnl)"=FALSE ("x/y scan")) -> ()  [unwired: 2 in, 2 out]
                  }
                }
              }
            }
          }
          event "XautoOD": Value Change {
            n2922 = event-data() -> ()  [unwired: 1 in, 1 out]
            n2923 = case shown="True" "XautoOD" {
              frame False {
              }
              frame True {
                n2924 = stacked-sequence {
                  frame #0 {
                    n2925 = Current VI's Path() -> (path=w6125:path)
                    n2926 = Strip Path(path=w6125) -> (stripped path=w6126:path)  [unwired: 1 out]
                    n2927 = Build Path(base path=w6126, name or relative path="subVIs\\Misc\\ChangeautoODs.vi") -> (appended path=w6124:path)
                    n2928 = call <vilib>:"Set Busy.vi"() -> ("error out"=w6122:errorcluster)  [unwired: 10 in, 1 out]
                    n2929 = Open VI Reference(type specifier VI Refnum (for type only)=refnum<vi> refnum, vi path=w6124, error in (no error)=w6122) -> (vi reference=w6117:refnum<vi>, error out=w6119:errorcluster)  [unwired: 3 in]
                    n2930 = call-by-ref "?"(reference=w6117, error in=w6119) -> (reference out=w6121:refnum<vi>, error out=w6120:errorcluster)  [unwired: 12 in]
                    n2931 = Close Reference(reference=w6121, error in (no error)=w6120) -> (error out=w6116:errorcluster)
                    "status 2" <- w6116
                    n2932 = call <vilib>:"Unset Busy.vi"("error in (no error)"=w6116) -> ()  [unwired: 10 in, 1 out]
                  }
                  frame #1 {
                    n2933 = property on="XautoOD" class="Bool (strict)"("Val(Sgnl)"=FALSE ("x/y scan")) -> ()  [unwired: 2 in, 2 out]
                  }
                }
              }
            }
          }
          event "SetMan": Value Change {
            n2934 = event-data() -> ()  [unwired: 1 in, 1 out]
            n2935 = case shown="True" "SetMan" {
              frame False {
              }
              frame True {
                n2936 = stacked-sequence {
                  frame #0 {
                    w6129 = u16 0 items=["Rectangle", "Circle", "Freeform Boundary", "Freeform Interior"] ("ROI Type")
                    n2937 = local write "ROI Type"(w6129) -> ()
                    n2938 = local read "Square pixels"() -> (w6135:bool)
                    n2939 = case shown="True" w6135 {
                      frame False {
                        n2940 = local read "square matrix"() -> (w6136:bool)
                        n2941 = case shown="False" w6136 {
                          frame False {
                            "ypixels ref" <- "ypixels"
                            "xpixels ref" <- "xpixels"
                          }
                          frame True {
                            n2942 = local read "xpixels"() -> (w6141:i32)
                            n2943 = local read "ypixels"() -> (w6140:i32)
                            n2944 = Max & Min(x=w6141, y=w6140) -> (max(x,y)=w6139:i32)  [unwired: 1 out]
                            n2945 = local write "xpixels ref"(w6139) -> ()
                            n2946 = local write "ypixels ref"(w6139) -> ()
                          }
                        }
                      }
                      frame True {
                        n2947 = local read "square matrix"() -> (w6142:bool)
                        n2948 = case shown="False" w6142 {
                          frame False {
                            n2949 = local read "Vxmax"() -> (w6156:dbl)
                            n2950 = local read "Vx-min"() -> (w6155:dbl)
                            n2951 = local read "Vy-max"() -> (w6151:dbl)
                            n2952 = local read "Vy-min"() -> (w6152:dbl)
                            n2953 = Subtract(x=w6151, y=w6152) -> (x-y=w6153:dbl)
                            n2954 = Subtract(x=w6156, y=w6155) -> (x-y=w6154:dbl)
                            n2955 = Absolute Value(x=w6153) -> (abs(x)=w6144:dbl)
                            n2956 = Absolute Value(x=w6154) -> (abs(x)=w6145:dbl)
                            n2957 = Divide(x=w6145, y=w6144) -> (x/y=w6150:dbl)
                            n2958 = Greater Or Equal?(x=w6145, y=w6144) -> (x >= y?=w6143:bool)
                            n2959 = local read "xpixels"() -> (w6149:i32)
                            n2960 = local read "ypixels"() -> (w6146:i32)
                            n2961 = case shown="False" w6143 {
                              tunnel: w6150 -> [w6161 w6164]
                              tunnel: w6149 -> [w6158 _]
                              tunnel: [w6158 w6163] -> w6148
                              tunnel: [w6157 w6162] -> w6147
                              tunnel: w6146 -> [_ w6162]
                              frame False {
                                n2962 = To Double Precision Float(number=w6158) -> (double precision float=w6160:dbl)
                                n2963 = Divide(x=w6160, y=w6161) -> (x/y=w6159:dbl)
                                n2964 = To Long Integer(number=w6159) -> (32bit integer=w6157:i32)
                              }
                              frame True {
                                n2965 = To Double Precision Float(number=w6162) -> (double precision float=w6166:dbl)
                                n2966 = Multiply(x=w6166, y=w6164) -> (x*y=w6165:dbl)
                                n2967 = To Long Integer(number=w6165) -> (32bit integer=w6163:i32)
                              }
                            }
                            n2968 = local write "ypixels ref"(w6147) -> ()
                            n2969 = local write "xpixels ref"(w6148) -> ()
                          }
                          frame True {
                          }
                        }
                      }
                    }
                    "Vx-max ref" <- "Vxmax"
                    "Vx-min ref" <- "Vx-min"
                    "Vy-max ref" <- "Vy-max"
                    "Vy-min ref" <- "Vy-min"
                    "Angle ref" <- "Angle"
                  }
                  frame #1 {
                    n2970 = property on="SetMan" class="Bool (strict)"("Val(Sgnl)"=FALSE ("Value (Signaling)")) -> ()  [unwired: 2 in, 2 out]
                  }
                }
              }
            }
          }
          event "SetMan 2": Value Change {
            n2971 = event-data() -> ()  [unwired: 1 in, 1 out]
            n2972 = case shown="True" "SetMan 2" {
              frame False {
              }
              frame True {
                n2973 = stacked-sequence {
                  frame #0 {
                    n2974 = local write "Vx-ref"("Vx") -> ()
                    n2975 = local write "Vy-ref"("Vy") -> ()
                  }
                  frame #1 {
                    n2976 = property on="SetMan 2" class="Bool (strict)"("Val(Sgnl)"=FALSE ("Value (Signaling)")) -> ()  [unwired: 2 in, 2 out]
                  }
                }
              }
            }
          }
          event "Reset Coords": Value Change {
            n2977 = event-data() -> ("NewVal"=w6172:bool)  [unwired: 1 in, 5 out]
            n2978 = case shown="True" w6172 {
              frame False {
              }
              frame True {
                n2979 = stacked-sequence {
                  frame #0 {
                    n2980 = local write "xpixels"(256 ("xpixels")) -> ()
                    n2981 = local write "ypixels"(256 ("ypixels")) -> ()
                    n2982 = local write "Vxmax"(9.0 ("Vx-max")) -> ()
                    n2983 = local write "Vx-min"(-9.0 ("Vx-min")) -> ()
                    n2984 = local write "Vy-max"(9.0 ("Vy-max")) -> ()
                    n2985 = local write "Vy-min"(-9.0 ("Vy-min")) -> ()
                    n2986 = local write "Angle"(0.0 ("Angle")) -> ()
                  }
                  frame #1 {
                    n2987 = property on="Reset Coords" class="Bool (strict)"("Value"=FALSE ("TROI")) -> ()  [unwired: 2 in, 2 out]
                  }
                }
              }
            }
          }
          event "TROI": Value Change {
            n2988 = event-data() -> ()  [unwired: 1 in, 1 out]
            n2989 = case shown="True" "TROI" {
              frame False {
              }
              frame True {
                n2990 = stacked-sequence {
                  frame #0 {
                    n2991 = local read "Vy-min ref"() -> (w6186:dbl)
                    n2992 = local read "Vy-max ref"() -> (w6185:dbl)
                    n2993 = local read "Vx-max ref"() -> (w6183:dbl)
                    n2994 = local read "Vx-min ref"() -> (w6184:dbl)
                    n2995 = local read "ypixels ref"() -> (w6188:i32)
                    n2996 = local read "xpixels ref"() -> (w6187:i32)
                    n2997 = local read "Angle ref"() -> (w6182:dbl)
                    n2998 = local write "Angle"(w6182) -> ()
                    n2999 = local write "xpixels"(w6187) -> ()
                    n3000 = local write "Vy-min"(w6186) -> ()
                    n3001 = local write "Vy-max"(w6185) -> ()
                    n3002 = local write "Vx-min"(w6184) -> ()
                    n3003 = local write "ypixels"(w6188) -> ()
                    n3004 = local write "Vxmax"(w6183) -> ()
                  }
                  frame #1 {
                    n3005 = property on="TROI" class="Bool (strict)"("Value"=FALSE ("TROI")) -> ()  [unwired: 2 in, 2 out]
                  }
                }
              }
            }
          }
          event "TROI 2": Value Change {
            n3006 = event-data() -> ()  [unwired: 1 in, 1 out]
            n3007 = case shown="True" "TROI 2" {
              frame False {
              }
              frame True {
                n3008 = stacked-sequence {
                  frame #0 {
                    n3009 = local read "Vx-ref"() -> (w6191:dbl)
                    n3010 = local read "Vy-ref"() -> (w6192:dbl)
                    n3011 = local write "Vx"(w6191) -> ()
                    n3012 = local write "Vy"(w6192) -> ()
                  }
                  frame #1 {
                    n3013 = property on="TROI 2" class="Bool (strict)"("Value"=FALSE ("TROI")) -> ()  [unwired: 2 in, 2 out]
                  }
                }
              }
            }
          }
          event "Square pixels": Value Change {
            n3014 = event-data() -> ()  [unwired: 1 in, 1 out]
            n3015 = case shown="True" "Square pixels" {
              frame False {
              }
              frame True {
                n3016 = property on="square matrix" class="Bool (strict)"("Value"=FALSE ("square matrix")) -> ()  [unwired: 2 in, 2 out]
                n3017 = property on="Square pixels" class="Bool (strict)"("Value"=TRUE ("square matrix")) -> ()  [unwired: 2 in, 2 out]
              }
            }
          }
          event "square matrix": Value Change {
            n3018 = event-data() -> ()  [unwired: 1 in, 1 out]
            n3019 = case shown="True" "square matrix" {
              frame False {
              }
              frame True {
                n3020 = property on="square matrix" class="Bool (strict)"("Value"=TRUE ("square matrix")) -> ()  [unwired: 2 in, 2 out]
                n3021 = property on="Square pixels" class="Bool (strict)"("Value"=FALSE ("square matrix")) -> ()  [unwired: 2 in, 2 out]
              }
            }
          }
          event "up", "downright", "down", "downleft", "right", "left", "upright", "upleft": Value Change {
            n3022 = event-data() -> ()  [unwired: 1 in, 6 out]
            n3023 = local read "downright"() -> (w6205:bool)
            n3024 = local read "downleft"() -> (w6207:bool)
            n3025 = local read "upright"() -> (w6203:bool)
            n3026 = local read "upleft"() -> (w6201:bool)
            n3027 = local read "down"() -> (w6206:bool)
            n3028 = local read "right"() -> (w6204:bool)
            n3029 = local read "left"() -> (w6208:bool)
            n3030 = local read "up"() -> (w6202:bool)
            n3031 = Compound Arithmetic op=OR(w6201, w6202, w6203, w6204, w6205, w6206, w6207, w6208) -> (w6200:bool)
            n3032 = case shown="True" w6200 {
              frame False {
              }
              frame True {
                n3033 = stacked-sequence {
                  frame #0 {
                    n3034 = local read "downright"() -> (w6210:bool)
                    n3035 = local read "downleft"() -> (w6212:bool)
                    n3036 = local read "BigSmall"() -> (w6209:bool)
                    n3037 = local read "upright"() -> (w6214:bool)
                    n3038 = local read "upleft"() -> (w6217:bool)
                    n3039 = local read "down"() -> (w6213:bool)
                    n3040 = local read "right"() -> (w6215:bool)
                    n3041 = local read "left"() -> (w6211:bool)
                    n3042 = local read "up"() -> (w6216:bool)
                    n3043 = call "movestageparams.vi"("command"="get") -> ("Params out"=w6220:T20)  [unwired: 1 in]
                    n3044 = Bundle By Name(cluster=w6220, "upleft"=w6217, "up"=w6216, "upright"=w6214, "right"=w6215, "downright"=w6210, "down"=w6213, "downleft"=w6212, "left"=w6211, "Bigsmall"=w6209) -> (w6221:T20)
                    n3045 = call "movestageparams.vi"("Params in"=w6221, "command"="set") -> ()  [unwired: 1 out]
                  }
                  frame #1 {
                    n3046 = disable-structure shown="Disabled" {
                      frame Disabled {
                        n3047 = call "configuration.vi"("command"="get") -> ("config out"=w6224:T11)  [unwired: 2 in, 1 out]
                        n3048 = in-place {
                          n3049 = in-place-cluster #45(w6224) -> ()  [unwired: 2 out]
                          n3050 = in-place-cluster #45("StageL"="StageL", "StageS"="StageS") -> (w6222:T11)
                        }
                        n3051 = call "configuration.vi"("config in"=w6222, "command"="set") -> ()  [unwired: 1 in, 2 out]
                      }
                      frame Enabled {
                      }
                    }
                  }
                  frame #2 {
                    n3052 = call "movestage.vi"() -> ()  [unwired: 12 in]
                  }
                  frame #3 {
                    w6228 = FALSE ("OK Button")
                    w6229 = FALSE ("OK Button")
                    n3053 = property on="down" class="Bool (strict)"("Value"=w6229) -> ()  [unwired: 2 in, 2 out]
                    n3054 = property on="up" class="Bool (strict)"("Value"=w6229) -> ()  [unwired: 2 in, 2 out]
                    n3055 = property on="right" class="Bool (strict)"("Value"=w6229) -> ()  [unwired: 2 in, 2 out]
                    n3056 = property on="left" class="Bool (strict)"("Value"=w6229) -> ()  [unwired: 2 in, 2 out]
                    n3057 = property on="upright" class="Bool (strict)"("Value"=w6228) -> ()  [unwired: 2 in, 2 out]
                    n3058 = property on="downleft" class="Bool (strict)"("Value"=w6228) -> ()  [unwired: 2 in, 2 out]
                    n3059 = property on="downright" class="Bool (strict)"("Value"=w6228) -> ()  [unwired: 2 in, 2 out]
                    n3060 = property on="upleft" class="Bool (strict)"("Value"=w6228) -> ()  [unwired: 2 in, 2 out]
                  }
                }
              }
            }
          }
          event "finite samples": Value Change {
            n3061 = event-data() -> ("NewVal"=w6230:bool)  [unwired: 1 in]
            n3062 = flat-sequence {
              tunnel: w6230 -> [w6231]
              frame #0 {
                n3063 = case shown="True" w6231 {
                  frame False {
                    w6232 = FALSE ("wavdet")
                    n3064 = property on="continuous" class="Bool (strict)"("Value"=TRUE ("continuous for display")) -> ()  [unwired: 2 in, 2 out]
                    n3065 = property on="wavdet" class="Bool (strict)"("Value"=w6232) -> ()  [unwired: 2 in, 2 out]
                    n3066 = property on="save\ndata" class="Bool (strict)"("Value"=w6232) -> ()  [unwired: 2 in, 2 out]
                    n3067 = property on="# of frames" class="DigNum (strict)"("DisabledEnum"=T7."Disabled and Grayed Out" ("Disabled")) -> ()  [unwired: 2 in, 2 out]
                    n3068 = property on="save\ndata" class="Bool (strict)"("DisabledEnum"=T7."Disabled and Grayed Out" ("Disabled")) -> ()  [unwired: 2 in, 2 out]
                    "Save tab" <- enum32{"withsave", "withoutsave"}."withsave" ("Save tab")
                  }
                  frame True {
                    w6239 = FALSE ("continuous for display")
                    n3069 = property on="continuous" class="Bool (strict)"("Value"=w6239) -> ()  [unwired: 2 in, 2 out]
                    n3070 = property on="wavdet" class="Bool (strict)"("Value"=w6239) -> ()  [unwired: 2 in, 2 out]
                    n3071 = local write "Save tab"(enum32{"withsave", "withoutsave"}."withsave" ("Save tab")) -> ()
